vi "Start Call.vi"(6 "Event References":T3, 7 "Configuration (Default)":T1={"Std Out Stream-Split RegExp Pattern"="\\n", "Std Err Stream-Split RegExp Pattern"="\\n", "ID"="", "Windows UTF8 Conversion"=enum."To OEM Code Page"}, 8 "error in":errorcluster, 9 "Working Directory (default <Not A Path> - System Default)":path=path "" caption="Working Directory", 10 "Arguments (Default: Empty)":string[](array[string]), 11 "Executable Path":path) -> (0 "error out":errorcluster, 3 "New ASE Handle":refnum<class "ase.lvclass">)   [LabVIEW 2020, in "ase.lvlib" / "ase.lvclass"]
doc: "<B>Start an Asynchronous System Executable Call</B>\n\nThe absolute path to the executable should be supplied.\n\nThe User Events References to generate the \"Did Launch\", \"Standard Output\", \"Standard Error\" and \"Did Exit\" events can be supplied or omitted as required. <B>Ensure that the event registration process for any User Events passed to this VI has already been undertaken</B>.\n\nArguments that are to be passed to the executable are specified in an array. Ensure that each argument specifier or value is in a different array element. E.g. to call the ping executable with the arguments \"-n 10 localhost\" use the element values [ -n, 10, localhost]. (See https://www.boost.org/doc/libs/1_87_0/doc/html/boost_process/v2.html for more details)\n\n\nThe configuration class allows for override of certain behaviours such as the regular expression used to match the breaks in the Standard Out and Standard Error to be specified.\n\nThis VI generates the following errors:\n-4601: Poorly formatted/incorrect Regular Expression supplied.\n-5691000: Internal Library Error. <Check Error Message for more details>\n-5691301: Unable to launch the executable. <Check Error Message for more details>\n-5691305: Executable paths parameter cannot be an empty value."
uses:
  ase.lvclass
  Event References.ctl
  Standard Output.ctl
  Standard Error.ctl
  Did Exit.ctl
  Configuration.ctl
  Windows UTF8 Conversion Mode.ctl
  ase.lvclass/ase.ctl
  a70fc713-9ee9-4497-bede-7e71c94245f2.vi
  Error Internal Library Implementation Error.vi
  bin/ase_32-3.dll
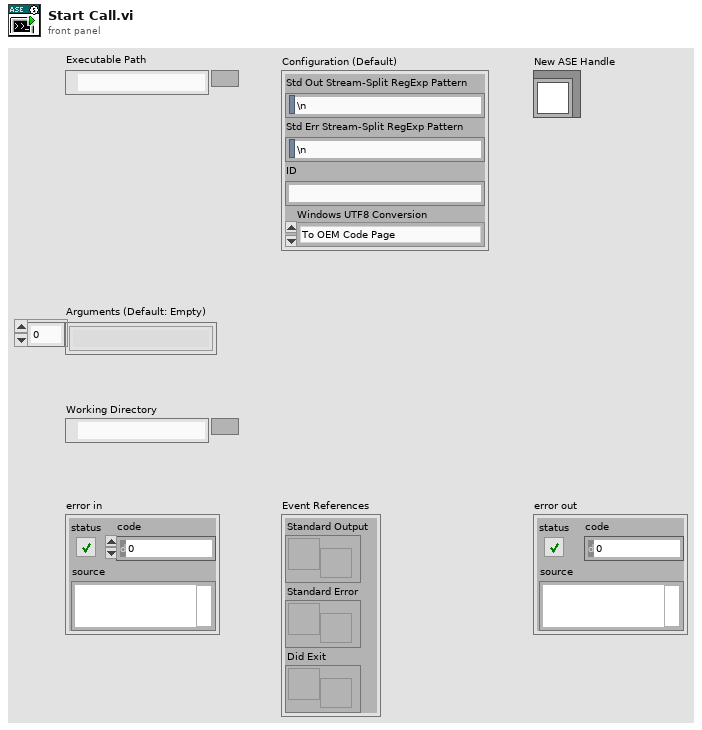
[diagram p1: front panel]
types:
  T1 = typedef "ase.lvlib/ase.lvclass/Configuration.ctl" = cluster{"Std Out Stream-Split RegExp Pattern":string, "Std Err Stream-Split RegExp Pattern":string, "ID":string, "Windows UTF8 Conversion":T2}
  T2 = typedef "ase.lvlib/ase.lvclass/Windows UTF8 Conversion Mode.ctl" = enum8{"None (Pass Through UTF8)", "To ACP Code Page", "To OEM Code Page"}
  T3 = typedef "ase.lvlib/ase.lvclass/Event References.ctl" = cluster{"Standard Output":refnum<user-event>, "Standard Error":refnum<user-event>, "Did Exit":refnum<user-event>}
  T4 = enum16{"Check Exe", "Check Version", "Check RegEx Std Out", "Check RegEx Std Err", "CLFN"}
  T5 = enum16{"Check Exe", "Check Version", "Check RegEx Std Out", "Check RegEx Std Err", "CLFN"}[]
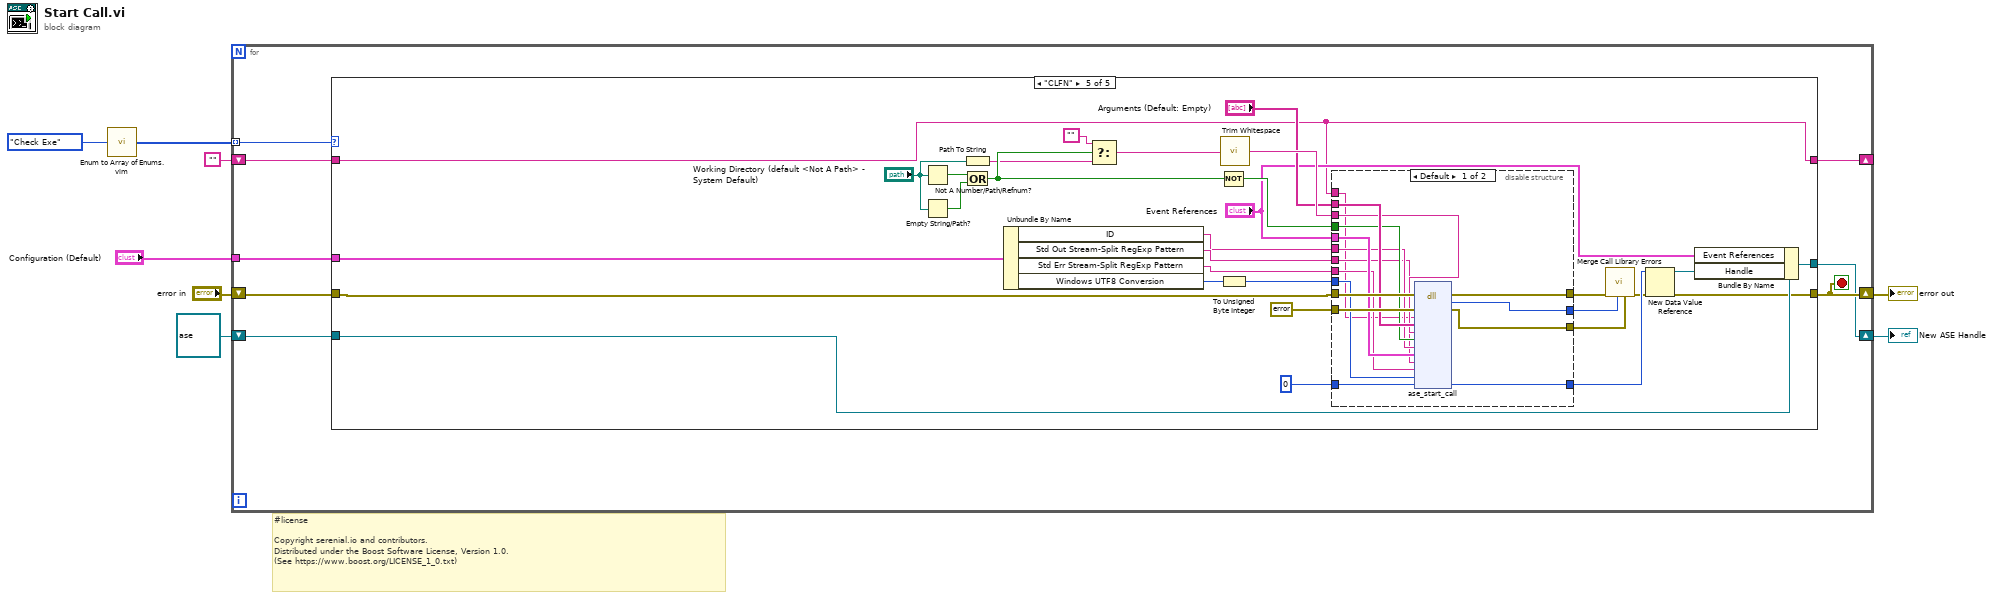
[diagram p0: block diagram]
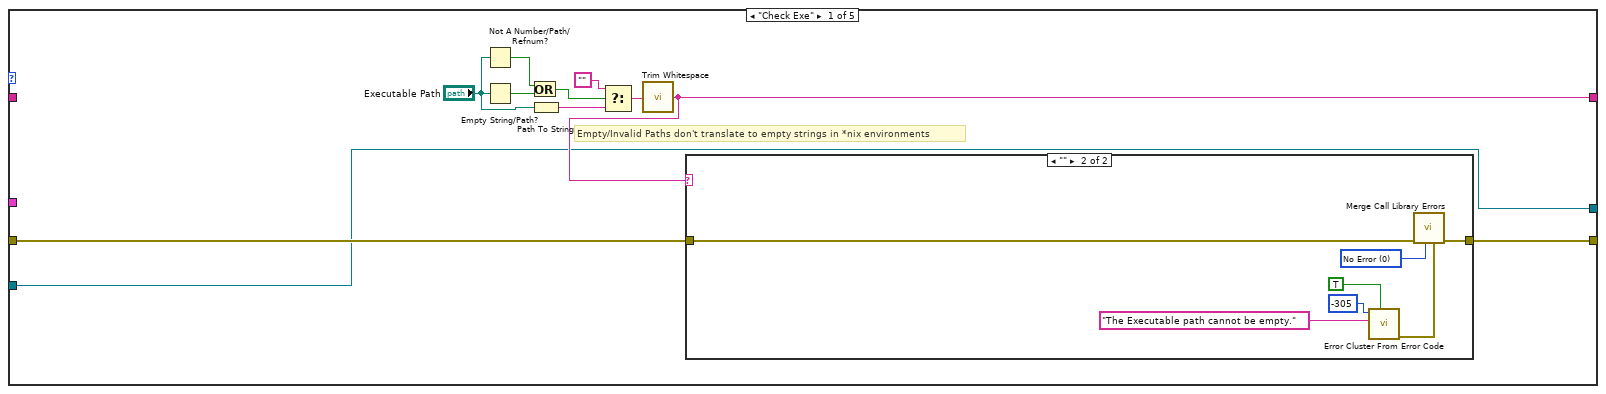
[diagram p2: hidden frame]
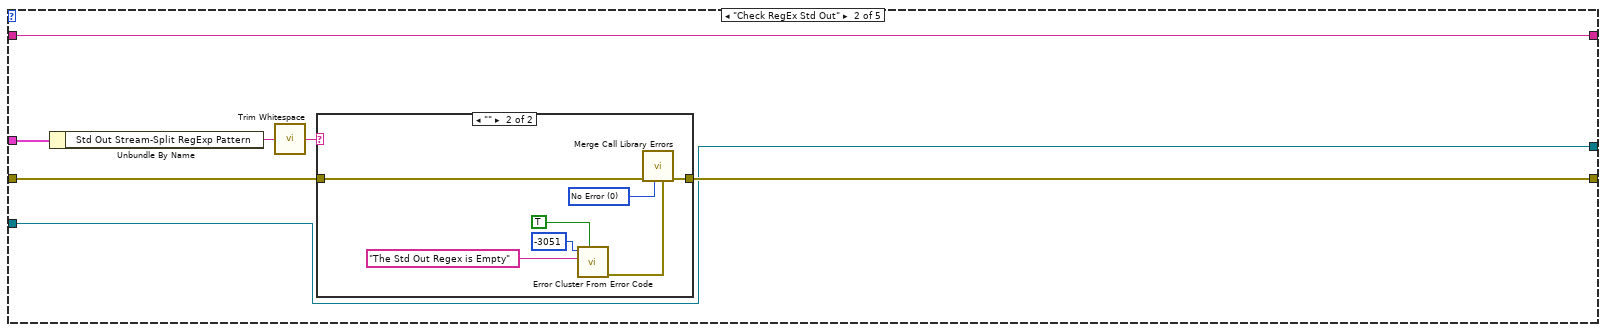
[diagram p4: hidden frame]
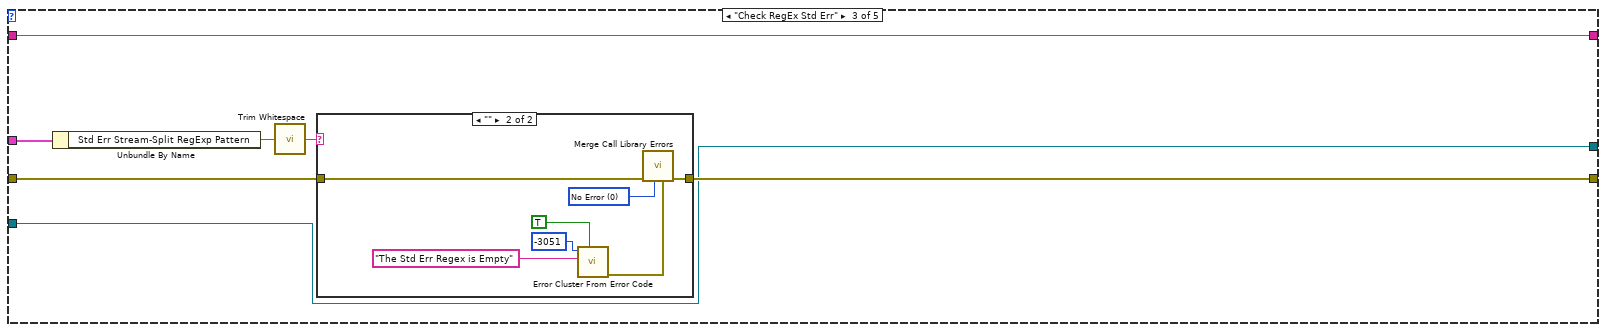
[diagram p6: hidden frame]
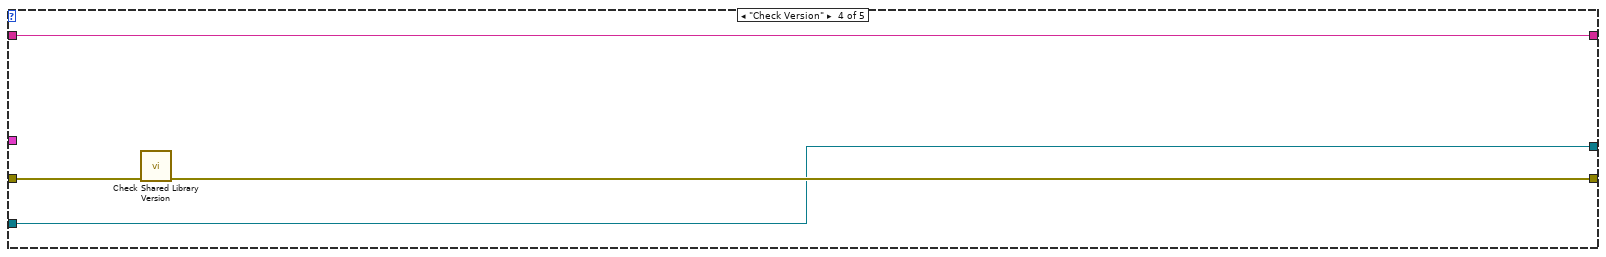
[diagram p8: hidden frame]
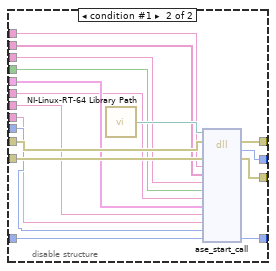
[diagram p9: hidden frame]
diagram:
  # "#license\n\nCopyright serenial.io and contributors.\nDistributed under the Boost Software License, Version 1.0.\n(See https://www.boost.org/LICENSE_1_0.txt)"
  n1 = call "Enum to Array of Enums.vim"("enum"=T4."Check Exe") -> ("array of enums"=w7:T5)
  n2 = for {
    tunnel: w7 -> [w16] mode=indexing
    shift-right: [w15] -> _
    shift-left: "" -> [w14]
    shift-right: [w12] -> w2
    shift-left: "error in" -> [w13]
    tunnel: "Configuration (Default)" -> [w11]
    shift-right: [w9] -> w3
    shift-left: refnum<class "ase.lvclass"> refnum ("serenial.io-ase.lvlib:ase.lvclass") -> [w10]
    stop <- w12 stop-if-true
    n3 = case shown="\"CLFN\"" w16 {
      tunnel: [w21 w42 w57 w67 w70] -> w15
      tunnel: w14 -> [_ w42 w57 w67 w70]
      tunnel: w13 -> [w20 w39 w54 w69 w73]
      tunnel: [w19 w38 w53 w68 w72] -> w12
      tunnel: w11 -> [_ w41 w56 _ w71]
      tunnel: w10 -> [w17 w36 w51 w66 w77]
      tunnel: [w17 w36 w51 w66 w74] -> w9
      frame "Check Exe" {
        # "Empty/Invalid Paths don't translate to empty strings in *nix environments"
        n4 = Not A Number/Path/Refnum?(number/path/refnum="Executable Path") -> (NaN/Path/Refnum?=w24:bool)
        n5 = Empty String/Path?(string/path="Executable Path") -> (empty?=w23:bool)
        n6 = Or(x=w24, y=w23) -> (x .or. y?=w25:bool)
        n7 = Path To String(path="Executable Path") -> (string=w26:string)
        n8 = Select(t="" ("Empty String Constant"), s=w25, f=w26) -> (s? t:f=w27:string)
        n9 = call "Trim Whitespace.vi"("Input"=w27) -> ("Output"=w21:string)
        n10 = case shown="\"\"" w21 {
          tunnel: w20 -> [w28 w32]
          tunnel: [w28 w30] -> w19
          frame Default {
          }
          frame "" {
            w31 = 0 items=["No Error", "mArgsErr", "mZoneErr", "mFullErr"] ("Error Code")
            n11 = call <vilib>:"Error Cluster From Error Code.vi"("show call chain? (False)"=TRUE, "error message (\"\")"="The Executable path cannot be empty." ("error message (\"\")"), "error code (0)"=-305) -> ("error out"=w33:errorcluster)  [unwired: 6 in]
            n12 = call "Merge Call Library Errors.vi"("Library Call Returned Error"=w33, "Error Code"=w31, "error in"=w32) -> ("error IO"=w30:errorcluster)  [unwired: 8 in]
          }
        }
      }
      frame "Check RegEx Std Out" {
        n13 = Unbundle By Name(w41) -> ("Std Out Stream-Split RegExp Pattern"=w40:string)
        n14 = call "Trim Whitespace.vi"("Input"=w40) -> ("Output"=w37:string)
        n15 = case shown="\"\"" w37 {
          tunnel: w39 -> [w43 w47]
          tunnel: [w43 w45] -> w38
          frame Default {
          }
          frame "" {
            w46 = 0 items=["No Error", "mArgsErr", "mZoneErr", "mFullErr"] ("Error Code")
            n16 = call <vilib>:"Error Cluster From Error Code.vi"("show call chain? (False)"=TRUE, "error message (\"\")"="The Std Out Regex is Empty" ("error message (\"\")"), "error code (0)"=-3051) -> ("error out"=w48:errorcluster)  [unwired: 6 in]
            n17 = call "Merge Call Library Errors.vi"("Library Call Returned Error"=w48, "Error Code"=w46, "error in"=w47) -> ("error IO"=w45:errorcluster)  [unwired: 8 in]
          }
        }
      }
      frame "Check RegEx Std Err" {
        n18 = Unbundle By Name(w56) -> ("Std Err Stream-Split RegExp Pattern"=w55:string)
        n19 = call "Trim Whitespace.vi"("Input"=w55) -> ("Output"=w52:string)
        n20 = case shown="\"\"" w52 {
          tunnel: w54 -> [w58 w62]
          tunnel: [w58 w60] -> w53
          frame Default {
          }
          frame "" {
            w61 = 0 items=["No Error", "mArgsErr", "mZoneErr", "mFullErr"] ("Error Code")
            n21 = call <vilib>:"Error Cluster From Error Code.vi"("show call chain? (False)"=TRUE, "error message (\"\")"="The Std Err Regex is Empty" ("error message (\"\")"), "error code (0)"=-3051) -> ("error out"=w63:errorcluster)  [unwired: 6 in]
            n22 = call "Merge Call Library Errors.vi"("Library Call Returned Error"=w63, "Error Code"=w61, "error in"=w62) -> ("error IO"=w60:errorcluster)  [unwired: 8 in]
          }
        }
      }
      frame "Check Version" {
        n23 = call "Check Shared Library Version.vi"("error in"=w69) -> ("error out"=w68:errorcluster)  [unwired: 9 in, 1 out]
      }
      frame "CLFN" {
        n24 = Not A Number/Path/Refnum?(number/path/refnum="Working Directory (default <Not A Path> - System Default)") -> (NaN/Path/Refnum?=w90:bool)
        n25 = Empty String/Path?(string/path="Working Directory (default <Not A Path> - System Default)") -> (empty?=w89:bool)
        n26 = Path To String(path="Working Directory (default <Not A Path> - System Default)") -> (string=w91:string)
        n27 = Or(x=w90, y=w89) -> (x .or. y?=w93:bool)
        n28 = Unbundle By Name(w71) -> ("ID"=w96:string, "Std Out Stream-Split RegExp Pattern"=w97:string, "Std Err Stream-Split RegExp Pattern"=w98:string, "Windows UTF8 Conversion"=w99:T2)
        n29 = Select(t="" ("Empty String Constant"), s=w93, f=w91) -> (s? t:f=w92:string)
        n30 = Not(x=w93) -> (.not. x?=w94:bool)
        n31 = To Unsigned Byte Integer(number=w99) -> (unsigned 8bit integer=w95:u8)
        n32 = call "Trim Whitespace.vi"("Input"=w92) -> ("Output"=w88:string)
        n33 = disable-structure "Conditional Disable Structure" shown="Default" {
          disable-tunnel: w73 -> [w114 w131]
          disable-tunnel: errorcluster {"status"=FALSE, "code"=0, "source"=""} ("error in (no error)") -> [w115 w130]
          disable-tunnel: u64 0 ("ASE interface pointer") -> [w100 w125]
          disable-tunnel: w88 -> [w112 w128]
          disable-tunnel: "Event References" -> [w110 w120]
          disable-tunnel: "Arguments (Default: Empty)" -> [w113 w129]
          disable-tunnel: w94 -> [w111 w127]
          disable-tunnel: w95 -> [w109 w126]
          disable-tunnel: [w108 w124] -> w86
          disable-tunnel: [w107 w123] -> w83
          disable-tunnel: [w106 w121] -> w84
          disable-tunnel: [w105 w122] -> w85
          disable-tunnel: w96 -> [w104 w118]
          disable-tunnel: w97 -> [w103 w117]
          disable-tunnel: w98 -> [w102 w116]
          disable-tunnel: w70 -> [w101 w119]
          frame condition #0 (active) {
            n34 = dll-call lib="C:/serenial/lib/asynchronous-system-exec/LabVIEW/ase/ase/bin/ase_*-3.*" fn="ase_start_call" ("AsyncSystemExec*.*:wrapperVersion")(error in=w114, "Error Out"=w115, "exe"=w101, "arguments"=w113, "working_directory"=w112, "use_working_directory"=w111, "id"=w104, "event_refs"=w110, "std_out_regex"=w103, "std_err_regex"=w102, "utf8-conversion"=w109, "handle"=w100) -> (error out=w107:errorcluster, "Error Code"=w106:i32, "Error Out"=w105:errorcluster, "handle"=w108:u64)  [unwired: 11 in, 1 out]
          }
          frame condition #1 {
            n35 = call "NI-Linux-RT-64 Library Path.vi"() -> ("Path"=w132:path)
            n36 = dll-call lib="?" fn="ase_start_call" ("AsyncSystemExec*.*:wrapperVersion")(path in=w132, error in=w131, "Error Out"=w130, "exe"=w119, "arguments"=w129, "working_directory"=w128, "use_working_directory"=w127, "id"=w118, "event_refs"=w120, "std_out_regex"=w117, "std_err_regex"=w116, "utf8-conversion"=w126, "handle"=w125) -> (error out=w123:errorcluster, "Error Code"=w121:i32, "Error Out"=w122:errorcluster, "handle"=w124:u64)  [unwired: 10 in, 1 out]
          }
        }
        n37 = call "Merge Call Library Errors.vi"("Library Call Returned Error"=w85, "Error Code"=w84, "error in"=w83) -> ("error IO"=w82:errorcluster)  [unwired: 8 in]
        n38 = New Data Value Reference(data value=w86, error in=w82) -> (data value reference=w75:refnum<data-value>, error out=w72:errorcluster)
        n39 = Bundle By Name(cluster=w77, "Event References"="Event References", "Handle"=w75) -> (w74:refnum<class "ase.lvclass">)
      }
    }
  }
  "error out" <- w2
  "New ASE Handle" <- w3
